vi "emi_is IP Address.vi"(7 "IP Address":string) -> (8 "IP Address?":bool)   [LabVIEW 2010]
doc: "Verify that strign is a valid IP adress. Four numbers between 0 and 255 seperated by \".\". First number can not be 0.\n\nReentrant Subroutine for throughput"
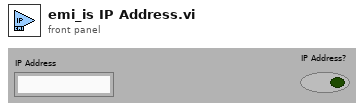
[diagram p1: front panel]
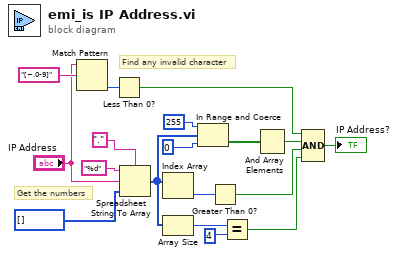
[diagram p0: block diagram]
diagram:
  # "Get the numbers"
  # "Find any invalid character"
  n1 = Match Pattern(string="IP Address", regular expression="[~.0-9]") -> (offset past match=w17:i32)  [unwired: 1 in, 3 out]
  n2 = Less Than 0?(x=w17) -> (x < 0?=w6:bool)
  n3 = Spreadsheet String To Array(delimiter (Tab)=".", format string="%d", spreadsheet string="IP Address", array type (2D Dbl)=i32[] []) -> (array=w1:i32[])
  n4 = Index Array(array=w1) -> (element=w9:i32)  [unwired: 1 in]
  n5 = Array Size(array=w1) -> (size(s)=w8:i32)
  n6 = In Range and Coerce(upper limit=255, x=w1, lower limit=0) -> (In Range?=w10:bool[])  [unwired: 1 out]
  n7 = Greater Than 0?(x=w9) -> (x > 0?=w4:bool)
  n8 = Equal?(x=w8, y=4) -> (x = y?=w3:bool)
  n9 = And Array Elements(Boolean array=w10) -> (logical AND=w5:bool)
  n10 = Compound Arithmetic op=AND(w6, w5, w4, w3) -> (→"IP Address?":bool)
